vi "Gate Width.vi"(7 "Read Value? (F)":bool, 8 "error in (no error)":errorcluster, 9 "Gate Width (0.005E-6 s)":dbl=0.005 min=5e-09 max=0.9992 format="%#_4e", 10 "Gate (A)":T1, 11 "VISA resource name":refnum<visa-resource-name>) -> (0 "error out":errorcluster, 1 "Gate Width":dbl=5e-09 format="%#_4e", 3 "VISA resource name out":refnum<visa-resource-name>)   [LabVIEW 2013, in "SRS SR400.lvlib"]
doc: "<B>GW i { ,t }</B>\n\nThe GW command sets and reads the gate widths. i = 0 or 1 designates A gate or B gate and is required. If t is included, the selected gate width is set to t seconds where 0.005E-6 <= t <= 999.2E-3. The resolution is variable depending upon the 4 most significant digits of t.\n\n<B>4 most significant digits</B> <B>resolution in 4th digit</B>\n1000 to 2048 1 (1001,1002,1003,...)\n2048 to 4096 2\n4096 to 8192 4\n8192 to 9992 8 (8192,8200,8208,...)\n\nFor example, near 10.00 us, the allowed values of t are 9.984 us, 9.992 us, 10.00 us, 10.01 us, etc. Below 1.000 us, the resolution is 1 ns. Almost any value of t may be sent and the SR400 will round to the nearest allowed value. If t is absent, the selected gate width is returned. The gate width may be read and set regardless of the gate mode. If the mode is CW, the gate remains continuous. If the mode is FIXED or SCAN, the gate width is adjusted immediately.\n\n<B>NOTE</B>\nChanging the gate delay or width may cause some gates to be missed or shortened. Changing gate parameters while counting may therefore cause bad data to be collected. It is recommended that the counters be paused before changing gate values and then started again."
uses:
  <instrlib>/SRS SR400/SRS SR400.lvlib
  <instrlib>/SRS SR400/Public/Typedefs/Gate.ctl
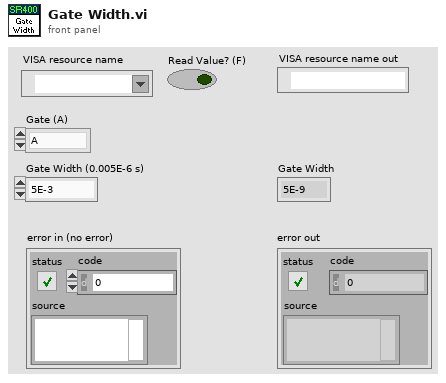
[diagram p1: front panel]
types:
  T1 = typedef "SRS SR400.lvlib/Gate.ctl" = enum16{"A", "B"}
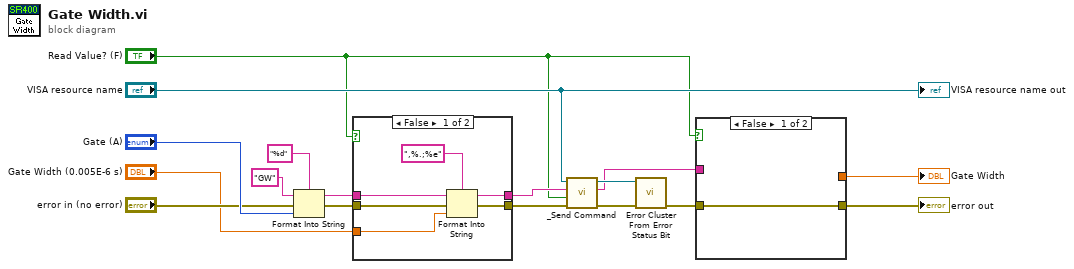
[diagram p0: block diagram]
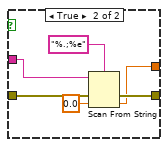
[diagram p2: hidden frame]
diagram:
  n1 = Format Into String(format string="%d", initial string="GW" ("command"), error in="error in (no error)", "Gate (A)") -> (resulting string=w14:string, error out=w15:errorcluster)
  n2 = case shown="False" "Read Value? (F)" {
    tunnel: w15 -> [w23 w24]
    tunnel: w14 -> [w18 w25]
    tunnel: "Gate Width (0.005E-6 s)" -> [w22 _]
    tunnel: [w20 w25] -> w10
    tunnel: [w19 w24] -> w9
    frame False {
      n3 = Format Into String(format string=",%.;%e", initial string=w18, error in=w23, w22) -> (resulting string=w20:string, error out=w19:errorcluster)
    }
    frame True {
    }
  }
  n4 = call <instrlib>:"_Send Command.vi"("error in (no error)"=w9, "Read Value? (F)"="Read Value? (F)", "Command"=w10, "VISA resource name"="VISA resource name") -> ("error out"=w6:errorcluster, "Response"=w2:string, "VISA resource name out"=w7:refnum<visa-resource-name>)  [unwired: 5 out]
  n5 = call <instrlib>:"Error Cluster From Error Status Bit.vi"("error in (no error)"=w6, "VISA resource name"=w7) -> ("error out"=w4:errorcluster)  [unwired: 8 in, 1 out]
  n6 = case shown="False" "Read Value? (F)" {
    tunnel: w4 -> [w26 w32]
    tunnel: [w26 w31] -> w3
    tunnel: w2 -> [_ w29]
    tunnel: [_ w28] -> w1
    frame False {
    }
    frame True {
      n7 = Scan From String(format string="%.;%e", input string=w29, error in=w32, default 1=0.0 ("default value 1")) -> (error out=w31:errorcluster, output 1=w28:dbl)  [unwired: 1 in, 2 out]
    }
  }
  "error out" <- w3
  "Gate Width" <- w1
  "VISA resource name out" <- "VISA resource name"
